vi "Build Tag.vi"(8 "Item":string, 9 "Section":string, 10 "Library Name":string, 11 "Project Name":string) -> (3 "Tag":string)   [LabVIEW 2019, in "Panther Dashboard.lvlib"]
uses:
  Panther Dashboard.lvlib
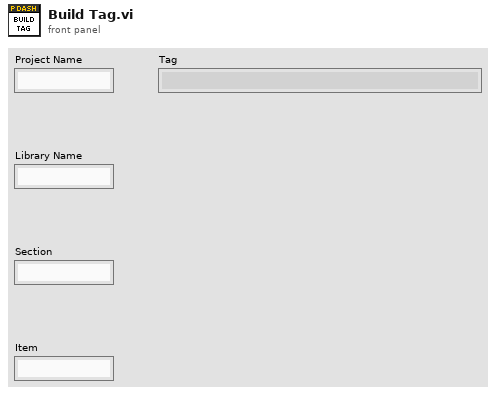
[diagram p1: front panel]
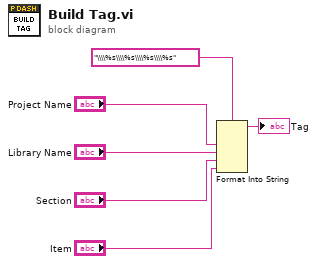
[diagram p0: block diagram]
diagram:
  n1 = Format Into String(format string="\\\\%s\\\\%s\\\\%s\\\\%s", "Project Name", "Library Name", "Section", "Item") -> (resulting string=→"Tag":string)  [unwired: 2 in, 1 out]
